vi "concatenate if path exists.vi"(10 "new path":path, 11 "paths in":path[](array[path])) -> (3 "paths out":path[](array[path]))   [LabVIEW 2013, in "PL_class cache.lvlib"]
uses:
  PL_class cache.lvlib
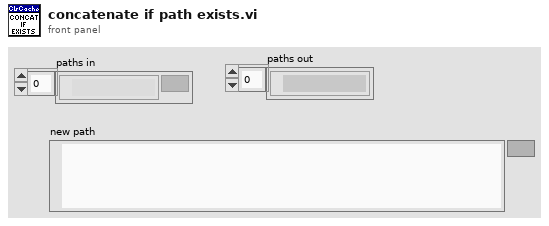
[diagram p1: front panel]
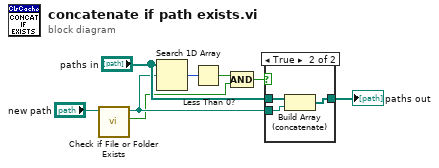
[diagram p0: block diagram]
diagram:
  n1 = call <vilib>:"Check if File or Folder Exists.vi"("path"="new path") -> ("file or folder exists?"=w4:bool, "dup path"=w5:path)  [unwired: 8 in, 1 out]
  n2 = Search 1D Array(1D array="paths in", element=w5) -> (index of element=w3:i32)  [unwired: 1 in]
  n3 = Less Than 0?(x=w3) -> (x < 0?=w2:bool)
  n4 = Compound Arithmetic op=AND(w2, w4) -> (w1:bool)
  n5 = case shown="True" w1 {
    tunnel: w5 -> [_ w12]
    tunnel: "paths in" -> [w9 w11]
    tunnel: [w9 w10] -> w8
    frame False {
    }
    frame True {
      n6 = Build Array (concatenate)(w11, w12) -> (w10:path[])
    }
  }
  "paths out" <- w8
